vi "isSubPanelReady.vi"(8 "error in (no error)":errorcluster, 11 "ActionEditor in":refnum<class "ActionEditor.lvclass">) -> (0 "error out":errorcluster, 2 "ready?":bool, 3 "ActionEditor out":refnum<class "ActionEditor.lvclass">)   [LabVIEW 2009, in "Views.lvlib" / "ScriptEditor.lvlib" / "ActionEditor.lvclass"]
uses:
  ActionEditor.lvclass
  ActionEditor.lvclass/ActionEditor.ctl
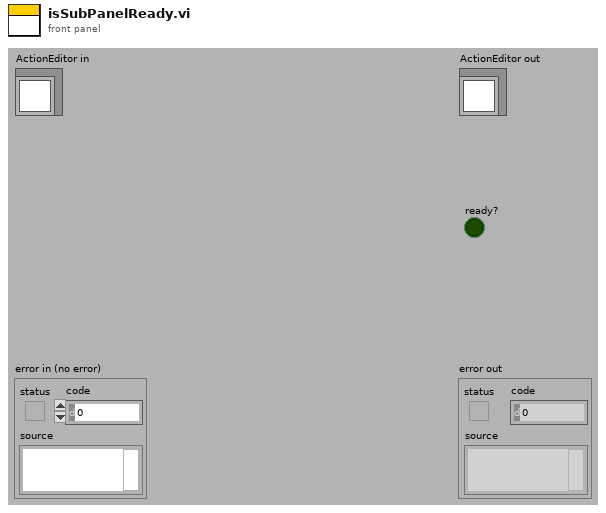
[diagram p1: front panel]
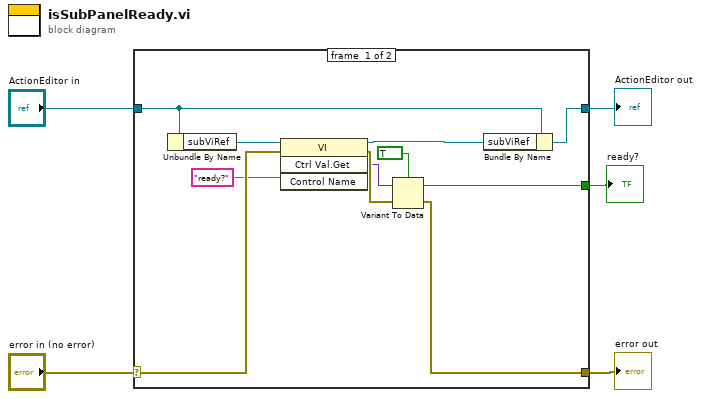
[diagram p0: block diagram]
diagram:
  n1 = case shown="No Error" "error in (no error)" {
    selector: "error in (no error)" -> [w15 w18]
    tunnel: [w9 w18] -> w4
    tunnel: [w6 w17] -> w2
    tunnel: "ActionEditor in" -> [w7 w17]
    tunnel: [w10 _] -> w1
    frame #0 {
      n2 = Unbundle By Name(w7) -> ("subViRef"=w16:refnum<vi>)
      n3 = invoke class="VI" method="Ctrl Val.Get"(reference=w16, error in=w15, "Control Name"="ready?") -> (reference out=w8:refnum<vi>, error out=w13:errorcluster, "Get Control Value Variant"=w12:variant)  [unwired: 1 in, 1 out]
      n4 = Variant To Data(error in=w13, Variant=w12, type=TRUE) -> (error out=w9:errorcluster, data=w10:bool)
      n5 = Bundle By Name(cluster=w7, "subViRef"=w8) -> (w6:refnum<class "ActionEditor.lvclass">)
    }
    frame #1 {
    }
  }
  "error out" <- w4
  "ActionEditor out" <- w2
  "ready?" <- w1
